vi "Test des thermistances - V2.vi"() -> ()   [LabVIEW 2020]
uses:
  <vilib>/Waveform/WDTOps.llb/WDT Append Waveforms DBL.vi
  <vilib>/Waveform/WDTFileIO.llb/Export Waveform To Spreadsheet File.vi
panel:
  in  "nom du périphérique":tag="Dev1"
  out "Graphique de la thermistance":waveform(dbl)(graph)
  in  "stop":bool
  # "Pour mon beau Philippe <3"
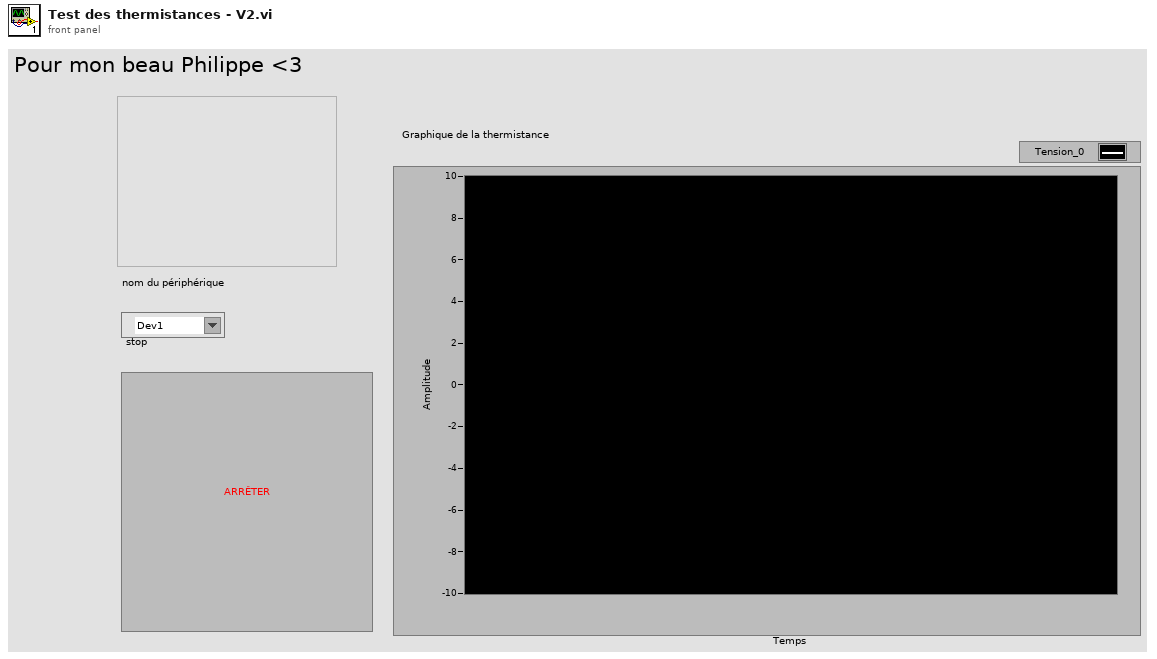
[diagram p1: front panel]
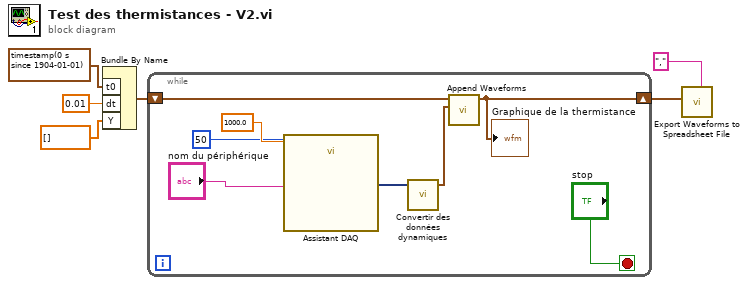
[diagram p0: block diagram]
diagram:
  n1 = Bundle By Name("t0"=timestamp(0 s since 1904-01-01), "dt"=0.01, "Y"=dbl[] []) -> (w3:waveform(dbl))  [unwired: 1 in]
  n2 = while {
    shift-right: [w10] -> w2
    shift-left: w3 -> [w12]
    stop <- "stop" stop-if-true
    n3 = call "Assistant DAQ"("vitesse"=1000.0, "nombre d'échantillons"=50, "nom du périphérique"="nom du périphérique") -> ("data"=w13:dynamicdata)  [unwired: 14 in, 2 out]
    n4 = call "Convertir des données dynamiques"("Dynamic Data Type"=w13) -> ("Waveform"=w11:waveform(dbl))  [unwired: 3 in]
    n5 = call-poly <vilib>:"Append Waveforms.vi"("waveform B"=w11, "waveform A"=w12) -> ("waveform out"=w10:waveform(dbl))  [unwired: 8 in, 1 out]
    "Graphique de la thermistance" <- w10
  }
  n6 = call-poly <vilib>:"Export Waveforms to Spreadsheet File.vi"("delimiter (Tab)"=",", "waveform"=w2) -> ()  [unwired: 8 in, 2 out]
